vi "Составление строки.vi"() -> ()   [LabVIEW 2017]
panel:
  out "hex integer string":string
  out "Длинна строки":i32
  in  "Число":dbl
  out "Результирующая строка":string
  in  "Окончание":string
  in  "Заголовок":string
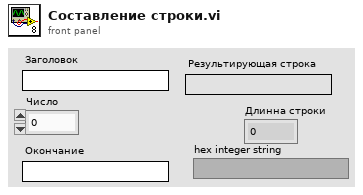
[diagram p1: front panel]
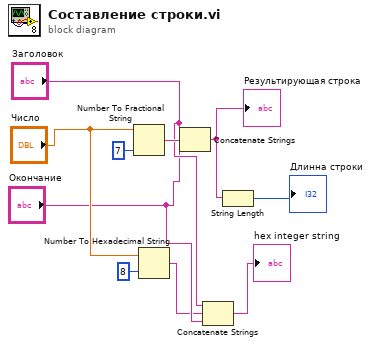
[diagram p0: block diagram]
diagram:
  n1 = Number To Fractional String(number="Число", precision (6)=i16 7) -> (F-format string=w9:string)  [unwired: 2 in]
  n2 = Number To Hexadecimal String(1:i16 8 ("width (-)"), 2:"Число") -> (0:w2:string)
  n3 = Concatenate Strings("Заголовок", w9, "Окончание") -> (w7:string)
  "Результирующая строка" <- w7
  n4 = Concatenate Strings("Заголовок", w2, "Окончание") -> (→"hex integer string":string)
  n5 = String Length(string=w7) -> (length=→"Длинна строки":i32)
